vi "Actor Core.vi"(8 "error in":errorcluster, 11 "Prime Panel in":refnum<class "Report Generator.lvclass">) -> (0 "error out":errorcluster, 3 "Actor out":refnum<class "Actor.lvclass">)   [LabVIEW 2023, in "Report Generator.lvlib" / "Report Generator.lvclass"]
doc: "Base class for the <b>Prime</b> subpanel.\nThis provides the basic implementation for show/hide operations.\n\n<b>Report Generator</b>\nThis routine monitors for events, and manages the event operations."
uses:
  Library/Report Generator.lvclass
  builds/Framework/Actor Framework.lvlibp/1abvi3w/vi.lib/ActorFramework/Actor/Actor.lvclass
  Report Generator Messages/Toggle Report Open Close Msg/Toggle Report Open Close Msg.lvclass/Toggle Report Open Close Msg.ctl
  builds/Framework/Actor Framework.lvlibp/1abvi3w/vi.lib/ActorFramework/Actor/Read Actor Label.vi
  builds/Framework/Actor Framework.lvlibp/1abvi3w/vi.lib/ActorFramework/Message Enqueuer/Enqueue.vi
  Report Generator Messages/Toggle Report Open Close Msg/Toggle Report Open Close Msg.lvclass
  builds/Main/Docking.lvlibp/Prime Panel/PrimeDock.lvclass
  Library/Report Generator.lvclass/Report Generator.ctl
  builds/Framework/Engine.lvlibp/Engine/Library/Engine.lvclass
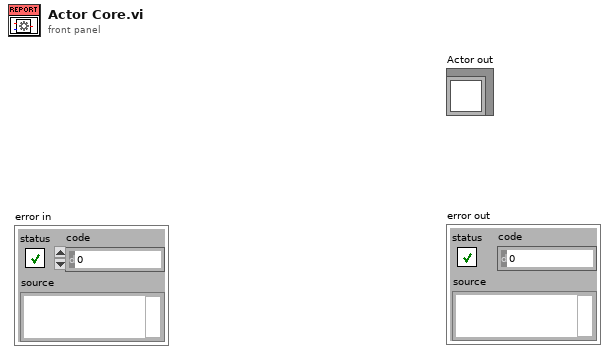
[diagram p1: front panel]
types:
  T1 = cluster{"Pnl Actor":refnum<event-registration>, "Event Registration Refnum":refnum<event-registration>}
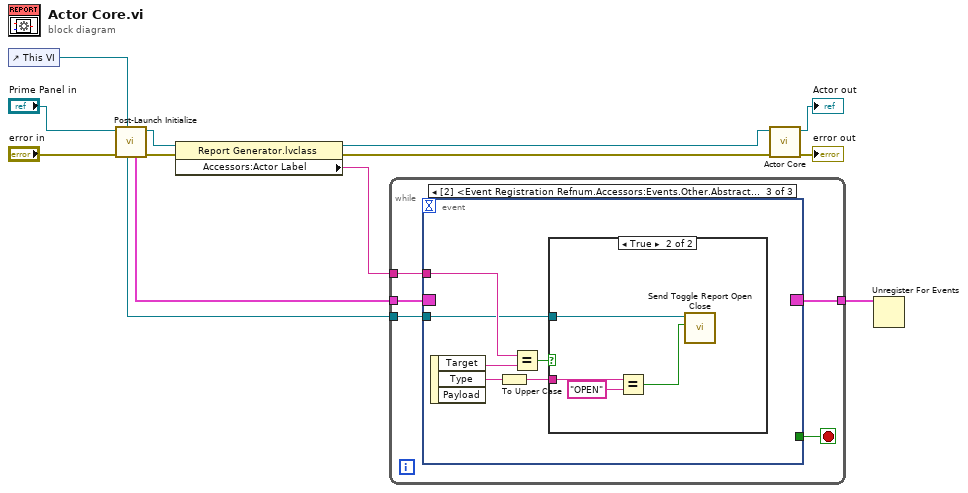
[diagram p0: block diagram]
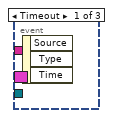
[diagram p2: hidden frame]
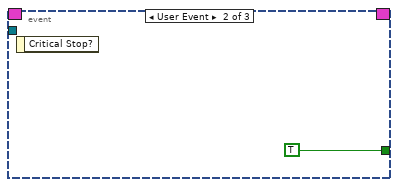
[diagram p3: hidden frame]
diagram:
  n1 = control-ref of="This VI"() -> (w8:refnum<vi>)
  n2 = call "Post-Launch Initialize.vi"("GUI Reference"=w8, "error in (no error)"="error in", "Engine in"="Prime Panel in") -> ("error out"=w10:errorcluster, "Engine out"=w3:refnum<class "Report Generator.lvclass">, "Registered Events"=w6:T1, "Self Enqueuer"=w5:refnum<class "Message Enqueuer.lvclass">)  [unwired: 5 in]
  n3 = property class="Report Generator.lvclass"(reference=w3, error in=w10) -> (reference out=w1:refnum<class "Report Generator.lvclass">, error out=w4:errorcluster, "Accessors:Actor Label"=w2:string)
  n4 = while {
    tunnel: [w18] -> w7
    tunnel: w6 -> [w17]
    tunnel: w5 -> [w15]
    tunnel: w2 -> [w14]
    stop <- w16 stop-if-true
    n5 = event shown="[2] <Event Registration Refnum.Accessors:Events.Other.AbstractMessage>: User Event" {
      selector: w17 -> [_ _ _]
      dyn-events: [_ _ _] -> w18
      timeout: _ -> [_ _ _]
      tunnel: [_ TRUE _] -> w16
      tunnel: w15 -> [_ _ w21]
      tunnel: w14 -> [_ _ w24]
      event Timeout {
        n6 = event-data() -> ()  [unwired: 1 in, 3 out]
      }
      event User Event {
        n7 = event-data() -> ()  [unwired: 1 in, 1 out]
      }
      event User Event {
        n8 = event-data() -> ("Target"=w25:string, "Type"=w22:string)  [unwired: 1 in, 1 out]
        n9 = To Upper Case(1:w22) -> (0:w20:string)
        n10 = Equal?(x=w24, y=w25) -> (x = y?=w23:bool)
        n11 = case shown="True" w23 {
          tunnel: w20 -> [_ w29]
          tunnel: w21 -> [_ w27]
          frame False {
          }
          frame True {
            n12 = Equal?(x=w29, y="OPEN") -> (x = y?=w26:bool)
            n13 = call "Send Toggle Report Open Close.vi"("Open"=w26, "Message Enqueuer"=w27) -> ()  [unwired: 8 in, 2 out]
          }
        }
      }
    }
  }
  n14 = call-parent "Actor Core.vi"("error in"=w4, "Prime Panel in"=w1) -> ("error out"=→"error out":errorcluster, "Actor out"=→"Actor out":refnum<class "Actor.lvclass">)  [unwired: 8 in]
  n15 = Unregister For Events(event registration refnum=w7) -> ()  [unwired: 1 in, 1 out]
